vi "ConvertCanTimestampToDateTimeStr.vi"(11 "Timestamp":dbl format="%<%I:%M:%S%3u %p\n%m/%d/%Y>T") -> (3 "Current Time and Date":string)   [LabVIEW 2018, in "Library-DataConvert.lvlib"]
uses:
  Library-DataConvert.lvlib
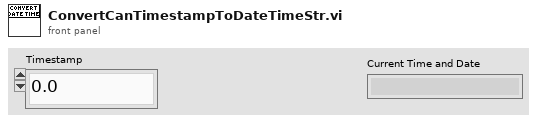
[diagram p1: front panel]
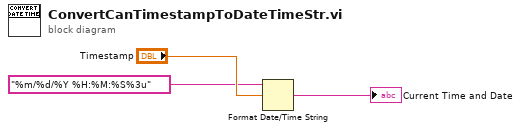
[diagram p0: block diagram]
diagram:
  n1 = Format Date/Time String(time format string (%c)="%m/%d/%Y %H:%M:%S%3u", seconds (now)="Timestamp") -> (date/time string=→"Current Time and Date":string)  [unwired: 1 in]
